vi "DialogEditClassIcon.vi"(0 "ClassWriter in":refnum<class "ClassWriter.lvclass">, 1 "ProjectItem Refnum":refnum<vi>, 5 "error in (no error)":errorcluster) -> (14 "ClassWriter out":refnum<class "ClassWriter.lvclass">, 19 "error out":errorcluster)   [LabVIEW 2016, in "ClassWriter.lvclass"]
uses:
  <resource>/Framework/Providers/Open_GDS/ClassProviders/Provider_BaseClassInterface/ClassWriter_class/ClassWriter.lvclass
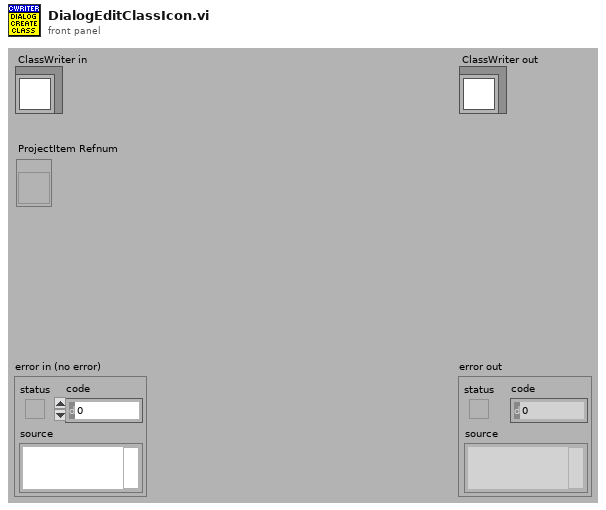
[diagram p1: front panel]
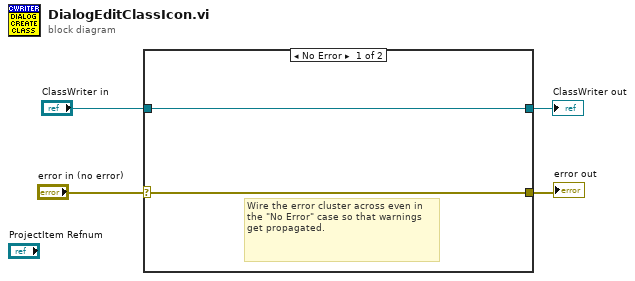
[diagram p0: block diagram]
diagram:
  n1 = case shown="No Error" "error in (no error)" {
    selector: "error in (no error)" -> [w5 w8]
    tunnel: [w5 w8] -> w3
    tunnel: [w6 w7] -> w1
    tunnel: "ClassWriter in" -> [w6 w7]
    frame No Error {
      # "Wire the error cluster across even in the \"No Error\" case so that warnings get propagated."
    }
    frame Error {
    }
  }
  "error out" <- w3
  "ClassWriter out" <- w1
